vi "ISX3_Example_Calibration.vi"() -> ()   [LabVIEW 2012, in "Sciospec ISX3 Impedance Analyzer.lvlib"]
uses:
  Sciospec ISX3 Impedance Analyzer.lvlib
panel:
  out "Load":bool
  out "ACK":bool
  out "Short":bool
  out "ACK":bool
  out "ACK":bool
  out "Open":bool
  out "ACK":bool
  out "CACK":bool
  out "ACK":bool
  out "ACK":bool
  out "CACK from ISX-3 to signal end of calibration":u8[](array[numeric])
  out "ACK for CACK":u8[](array[numeric])
  out "ACK Calibration Interaction":u8[](array[numeric])
  out "ACK for CACK":u8[](array[numeric])
  out "Calibration Interaction\nRequest for short":u8[](array[numeric])
  out "ACK for CACK":u8[](array[numeric])
  in  "Load Type":u8(ring)=1 items=["Resistance"=1, "Capacitator"=2]
  in  "Calibration Value":sgl
  in  "Next Calibration Step 2":bool
  out "Calibration Interaction\nRequest for load":u8[](array[numeric])
  in  "Next Calibration Step":bool
  in  "Next Calibration Step":bool
  out "Calibration Interaction\nRequest for open":u8[](array[numeric])
  out "ACK for Start Calibration":u8[](array[numeric])
  out "ACK for Load Setup":u8[](array[numeric])
  in  "Setup Slot":u8=1 min=1 step=1
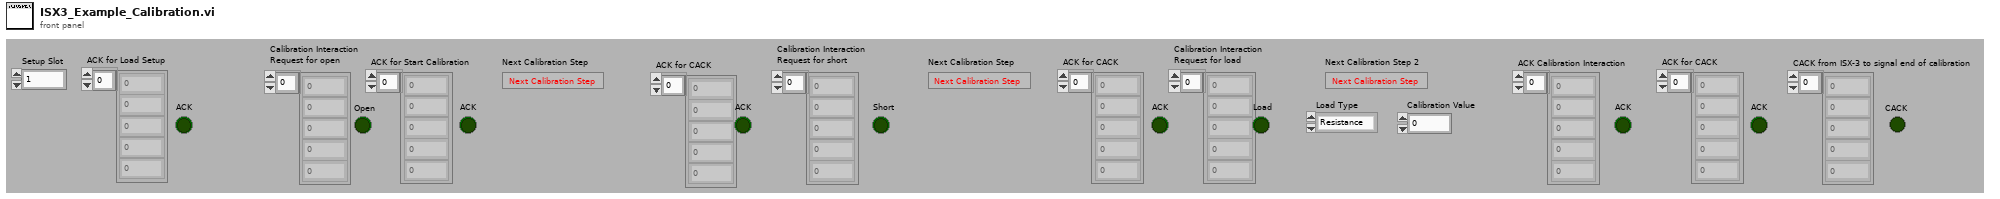
[diagram p1: front panel]
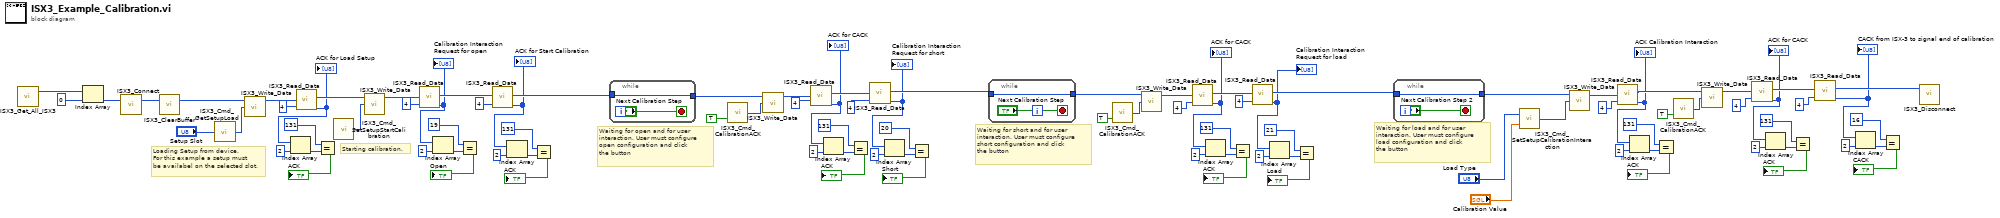
[diagram p0: block diagram]
diagram:
  # "Starting calibration."
  # "Loading Setup from device.\nFor this example a setup must\nbe availabel on the selected slot."
  # "Waiting for load and for user \ninteraction. User must configure \nload configuration and click\nthe button"
  # "Waiting for short and for user \ninteraction. User must configure \nshort configuration and click\nthe button"
  # "Waiting for open and for user \ninteraction. User must configure \nopen configuration and click\nthe button"
  n1 = call "ISX3_Get_All_ISX3.vi"() -> ("A list of FT_Handel where an ISX-3 is connected to.\nThis handle must be used for further interaction \nwith the USB interface."=w95:u32[])  [unwired: 2 in]
  n2 = Index Array(array=w95, index=u32 0) -> (element=w94:u32)
  n3 = call "ISX3_Connect.vi"("Connect to device with\nFT_Handle"=w94) -> ("Connected to device:"=w65:u32)  [unwired: 2 in]
  n4 = call "ISX3_ClearBuffer.vi"("Handle"=w65) -> ("Handle"=w64:u32)  [unwired: 1 in, 1 out]
  n5 = call "ISX3_Cmd_GetSetupLoad.vi"("Setup Slot"="Setup Slot") -> ("get Setup Load Cmd"=w93:u8[])
  n6 = call "ISX3_Write_Data.vi"("Data to Write"=w93, "FT_Handle"=w64) -> ("FT_Handle"=w91:u32)  [unwired: 2 in, 1 out]
  n7 = call "ISX3_Read_Data.vi"("FT_Handle"=w91, "Bytes To Read"=u32 4) -> ("Handle"=w89:u32, "Read Data"=w31:u8[])  [unwired: 2 in, 1 out]
  "ACK for Load Setup" <- w31
  n8 = Index Array(array=w31, index=2 ("Index")) -> (element=w33:u8)
  n9 = Equal?(x=u8 131, y=w33) -> (x = y?=→"ACK":bool)
  n10 = call "ISX3_Cmd_SetSetupStartCalibration.vi"() -> ("set Setup Start Calibration Cmd"=w88:u8[])  [unwired: 1 in]
  n11 = call "ISX3_Write_Data.vi"("Data to Write"=w88, "FT_Handle"=w89) -> ("FT_Handle"=w86:u32)  [unwired: 2 in, 1 out]
  n12 = call "ISX3_Read_Data.vi"("FT_Handle"=w86, "Bytes To Read"=u32 4) -> ("Handle"=w84:u32, "Read Data"=w26:u8[])  [unwired: 2 in, 1 out]
  "Calibration Interaction\nRequest for open" <- w26
  n13 = Index Array(array=w26, index=2 ("Index")) -> (element=w28:u8)
  n14 = Equal?(x=u8 19, y=w28) -> (x = y?=→"Open":bool)
  n15 = call "ISX3_Read_Data.vi"("FT_Handle"=w84, "Bytes To Read"=u32 4) -> ("Handle"=w83:u32, "Read Data"=w21:u8[])  [unwired: 2 in, 1 out]
  "ACK for Start Calibration" <- w21
  n16 = Index Array(array=w21, index=2 ("Index")) -> (element=w23:u8)
  n17 = Equal?(x=u8 131, y=w23) -> (x = y?=→"ACK":bool)
  n18 = while {
    tunnel: w83 -> [w97]
    tunnel: [w97] -> w73
    stop <- "Next Calibration Step" stop-if-true
  }
  n19 = call "ISX3_Cmd_CalibrationACK.vi"("ACK / NACK"=TRUE) -> ("ACK / NACK Calibration cmd"=w81:u8[])  [unwired: 1 in]
  n20 = call "ISX3_Write_Data.vi"("Data to Write"=w81, "FT_Handle"=w73) -> ("FT_Handle"=w68:u32)  [unwired: 2 in, 1 out]
  n21 = call "ISX3_Read_Data.vi"("FT_Handle"=w68, "Bytes To Read"=u32 4) -> ("Handle"=w67:u32, "Read Data"=w16:u8[])  [unwired: 2 in, 1 out]
  "ACK for CACK" <- w16
  n22 = Index Array(array=w16, index=2 ("Index")) -> (element=w18:u8)
  n23 = Equal?(x=u8 131, y=w18) -> (x = y?=→"ACK":bool)
  n24 = call "ISX3_Read_Data.vi"("FT_Handle"=w67, "Bytes To Read"=u32 4) -> ("Handle"=w66:u32, "Read Data"=w11:u8[])  [unwired: 2 in, 1 out]
  "Calibration Interaction\nRequest for short" <- w11
  n25 = Index Array(array=w11, index=2 ("Index")) -> (element=w13:u8)
  n26 = Equal?(x=u8 20, y=w13) -> (x = y?=→"Short":bool)
  n27 = while {
    tunnel: w66 -> [w99]
    tunnel: [w99] -> w78
    stop <- "Next Calibration Step" stop-if-true
  }
  n28 = call "ISX3_Cmd_CalibrationACK.vi"("ACK / NACK"=TRUE) -> ("ACK / NACK Calibration cmd"=w79:u8[])  [unwired: 1 in]
  n29 = call "ISX3_Write_Data.vi"("Data to Write"=w79, "FT_Handle"=w78) -> ("FT_Handle"=w70:u32)  [unwired: 2 in, 1 out]
  n30 = call "ISX3_Read_Data.vi"("FT_Handle"=w70, "Bytes To Read"=u32 4) -> ("Handle"=w69:u32, "Read Data"=w6:u8[])  [unwired: 2 in, 1 out]
  "ACK for CACK" <- w6
  n31 = Index Array(array=w6, index=2 ("Index")) -> (element=w8:u8)
  n32 = Equal?(x=u8 131, y=w8) -> (x = y?=→"ACK":bool)
  n33 = call "ISX3_Read_Data.vi"("FT_Handle"=w69, "Bytes To Read"=u32 4) -> ("Handle"=w77:u32, "Read Data"=w1:u8[])  [unwired: 2 in, 1 out]
  "Calibration Interaction\nRequest for load" <- w1
  n34 = Index Array(array=w1, index=2 ("Index")) -> (element=w3:u8)
  n35 = Equal?(x=u8 21, y=w3) -> (x = y?=→"Load":bool)
  n36 = while {
    tunnel: w77 -> [w101]
    tunnel: [w101] -> w74
    stop <- "Next Calibration Step 2" stop-if-true
  }
  n37 = call "ISX3_Cmd_SetSetupCalibrationInteraction.vi"("Calibration Value"="Calibration Value", "Load Type"="Load Type") -> ("set Setup Start Calibration Cmd"=w75:u8[])
  n38 = call "ISX3_Write_Data.vi"("Data to Write"=w75, "FT_Handle"=w74) -> ("FT_Handle"=w60:u32)  [unwired: 2 in, 1 out]
  n39 = call "ISX3_Read_Data.vi"("FT_Handle"=w60, "Bytes To Read"=u32 4) -> ("Handle"=w56:u32, "Read Data"=w46:u8[])  [unwired: 2 in, 1 out]
  "ACK Calibration Interaction" <- w46
  n40 = Index Array(array=w46, index=2 ("Index")) -> (element=w48:u8)
  n41 = Equal?(x=u8 131, y=w48) -> (x = y?=→"ACK":bool)
  n42 = call "ISX3_Cmd_CalibrationACK.vi"("ACK / NACK"=TRUE) -> ("ACK / NACK Calibration cmd"=w58:u8[])  [unwired: 1 in]
  n43 = call "ISX3_Write_Data.vi"("Data to Write"=w58, "FT_Handle"=w56) -> ("FT_Handle"=w55:u32)  [unwired: 2 in, 1 out]
  n44 = call "ISX3_Read_Data.vi"("FT_Handle"=w55, "Bytes To Read"=u32 4) -> ("Handle"=w53:u32, "Read Data"=w41:u8[])  [unwired: 2 in, 1 out]
  "ACK for CACK" <- w41
  n45 = Index Array(array=w41, index=2 ("Index")) -> (element=w43:u8)
  n46 = Equal?(x=u8 131, y=w43) -> (x = y?=→"ACK":bool)
  n47 = call "ISX3_Read_Data.vi"("FT_Handle"=w53, "Bytes To Read"=u32 4) -> ("Handle"=w52:u32, "Read Data"=w36:u8[])  [unwired: 2 in, 1 out]
  "CACK from ISX-3 to signal end of calibration" <- w36
  n48 = Index Array(array=w36, index=2 ("Index")) -> (element=w38:u8)
  n49 = Equal?(x=u8 16, y=w38) -> (x = y?=→"CACK":bool)
  n50 = call "ISX3_Disconnect.vi"("FT_Handle"=w52) -> ()  [unwired: 2 in]
